vi "ESC Pre Analysis Plugin.vi"() -> ()   [LabVIEW 2022 SP3]
uses:
  <vilib>/Analysis/baseanly.llb/Mean (DBL).vi
  Globals/Meas_global.vi
  <vilib>/measure/matone.llb/Extract Single Tone Information 1 Chan.vi
  <vilib>/measure/NI_MAPro.lvlib
  <vilib>/Analysis/NI_AALBase.lvlib
panel:
  in  "Blades/Poles":i32[](array[numeric])
  in  "Freq Channels":i32[](array[numeric])
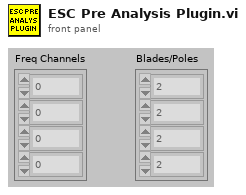
[diagram p1: front panel]
types:
  T1 = typedef "Analysis_info_cluster.ctl" = cluster{"Colour":u32, "Inst type":T2, "Inst name":string, "Symbol":string, "Code name":string, "Extra Info":string, "Inst Array":T3, "U":dbl, "u^2":dbl, "u^3":dbl, "u^4":dbl, "Skew_u":dbl, "Kurt_u":dbl, "Sd Error in Mean":dbl, "% u'/U":dbl, "X":dbl, "Y":dbl, "Z":dbl, "Timescale integral Estimate":dbl, "Sd Error in Variance":dbl, "Calib File":path, "Calib Constants":dbl[], "Output Position":bool, "Stats":enum16{"None", "Basic", "Full"}, "Av Sampling Rate":dbl, "Av No of Samples":dbl, "Total Meas Time (s)":dbl, "OrigChName":string, "Max value":dbl, "Min value":dbl, "Req Sample Rate Hz":dbl, "Sync Delay Time (s)":dbl, "Ch No":i16, "Device":string, "Use Latest Calib":bool, "Port":string, "Metadata Ch Names":string[], "Metadata Ch Values":string[], "Label":string, "chState":T4, "Point Drift":dbl, "inputConfig":string}
  T2 = typedef "Inst_type.ctl" = enum16{"Raw voltage", "Raw with zero offsetting", "Propeller anemometer", "Pressure Transducer", "Pitot-static tube", "Hot wire", "Cross wire 1", "Cross wire 2", "Generic Linear", "Generic Polynomial", "Generic BackPoly", "Fast FID", "Thermocouple", "Cold wire", "Pulsed Wire", "LDA Vel", "LDA Tran time", "LDA Arr time", "Microphone"}
  T3 = typedef "Instrument_Array.ctl" = enum16{"PWA", "LDA", "Analogue"}
  T4 = typedef "channelState.ctl" = enum32{"No Selection", "Solo", "Mute"}
  T5 = typedef "Setup.ctl" = enum16{"Run Program", "Show Setup", "Save Current Setup", "Setup Front Panel"}
  T6 = typedef "Time_Trace_Cluster.ctl" = cluster{"Weighting":dbl[], "Voltage":dbl[], "Eng Values":dbl[]}
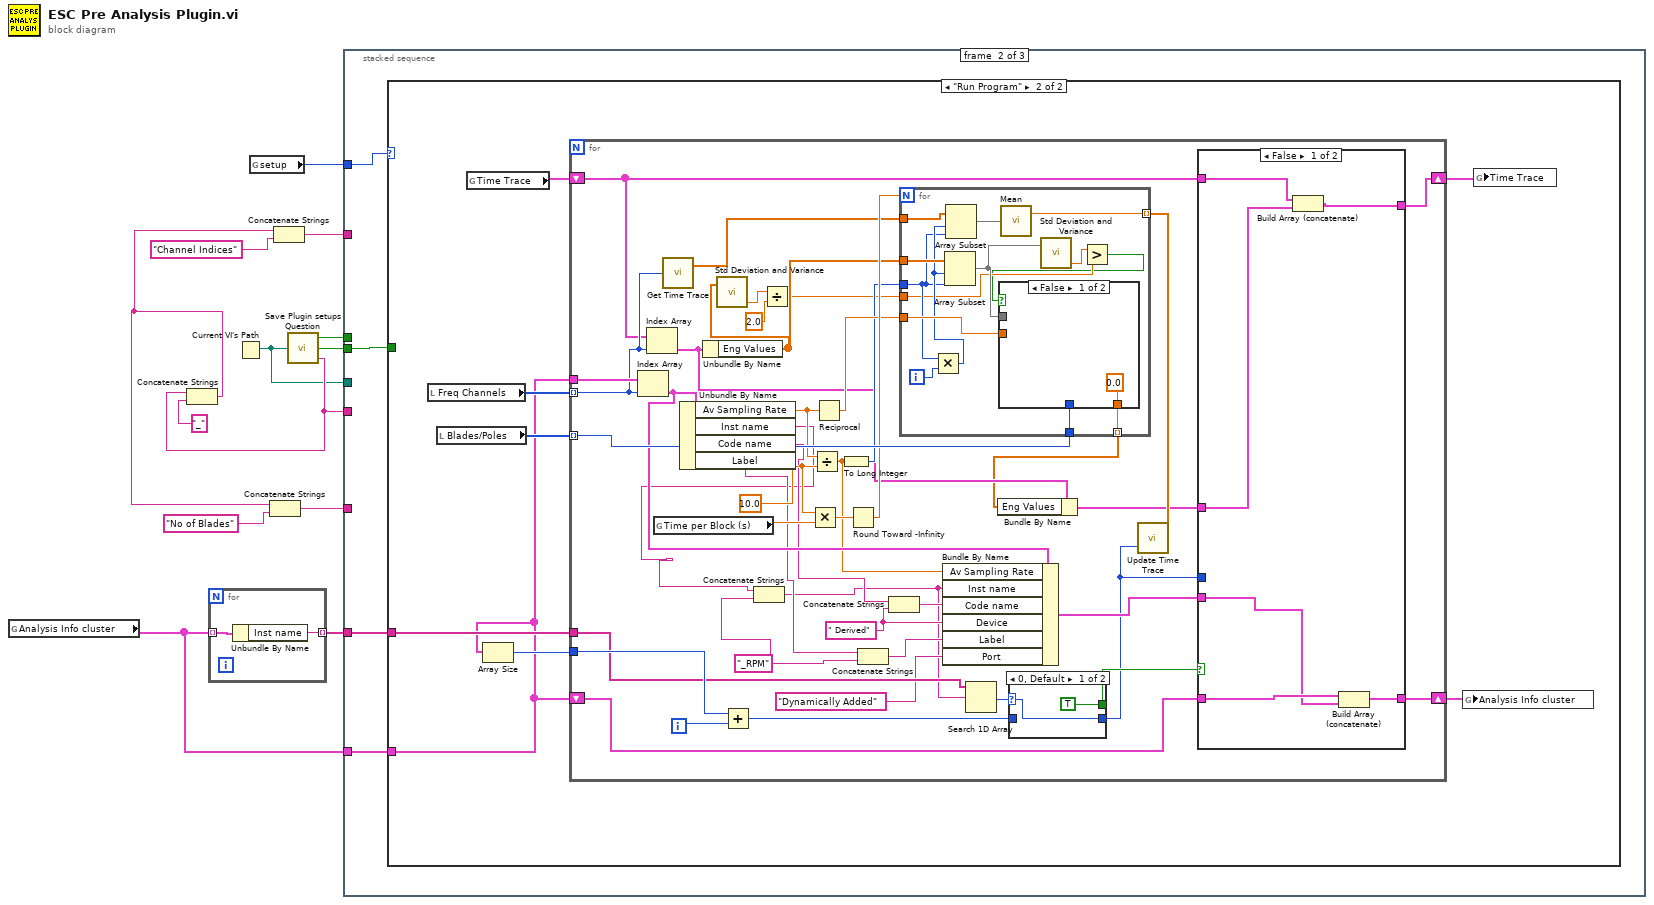
[diagram p0: block diagram]
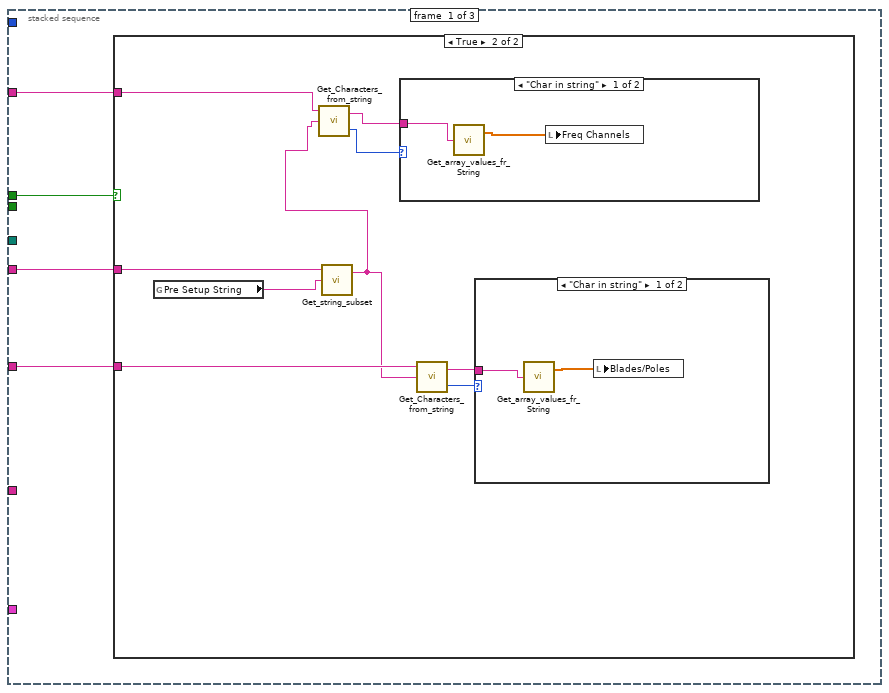
[diagram p2: hidden frame]
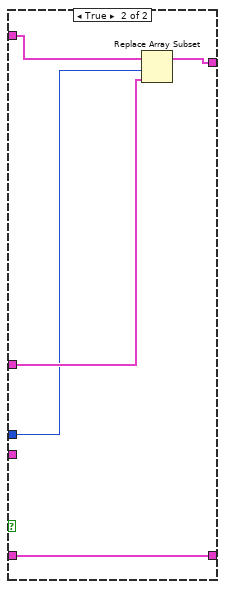
[diagram p7: hidden frame]
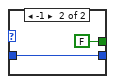
[diagram p8: hidden frame]
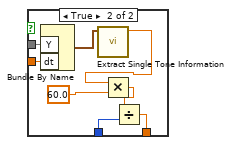
[diagram p9: hidden frame]
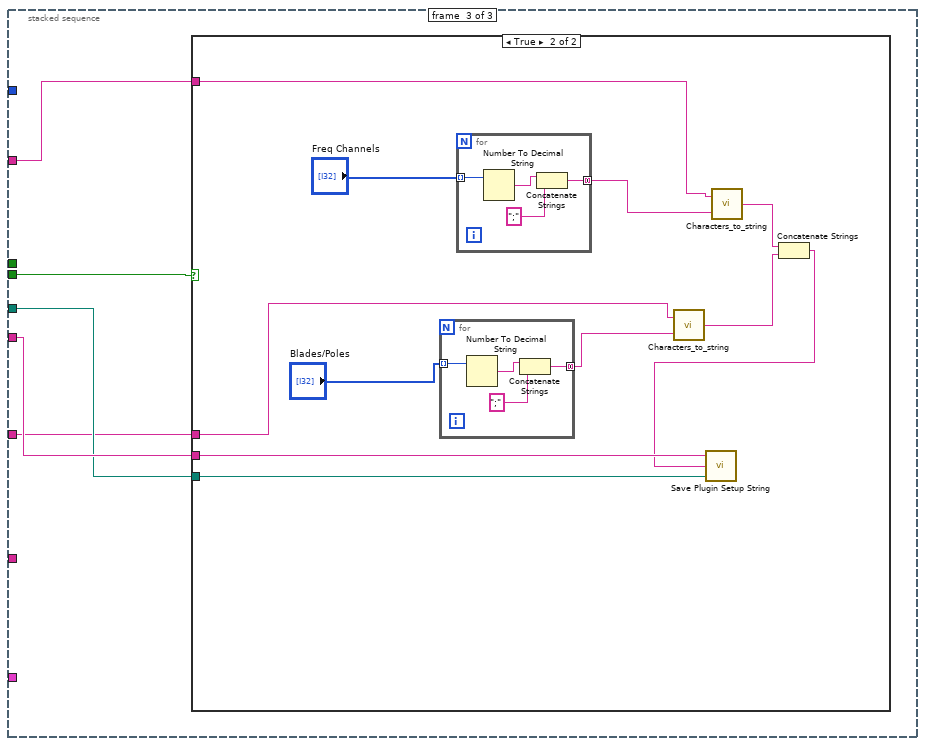
[diagram p10: hidden frame]
diagram:
  n1 = global read "Meas_global.vi" "Analysis Info cluster"() -> (w2:T1[])
  n2 = for {
    tunnel: w2 -> [w15] mode=indexing
    tunnel: [w14] -> w1 mode=indexing
    n3 = Unbundle By Name(w15) -> ("Inst name"=w14:string)
  }
  n4 = Current VI's Path() -> (path=w7:path)
  n5 = global read "Meas_global.vi" "setup"() -> (w3:T5)
  n6 = call "Save Plugin setups Question.vi"("VI path"=w7) -> ("Load Plugin Setup"=w13:bool, "Save Plugin Setup"=w8:bool, "Plugin_Label"=w9:string)
  n7 = Concatenate Strings(w9, "_" ("string")) -> (w5:string)
  n8 = Concatenate Strings(w5, "No of Blades" ("Label for value")) -> (w4:string)
  n9 = Concatenate Strings(w5, "Channel Indices" ("Label for value")) -> (w10:string)
  n10 = stacked-sequence {
    tunnel: w13 -> [w19 _ _]
    tunnel: w10 -> [w18 _ w127]
    tunnel: w9 -> [w17 _ w128]
    tunnel: w8 -> [_ w35 w129]
    tunnel: w7 -> [_ _ w126]
    tunnel: w4 -> [w16 _ w125]
    tunnel: w3 -> [_ w36 _]
    tunnel: w2 -> [_ w34 _]
    tunnel: w1 -> [_ w33 _]
    frame #0 {
      n11 = case shown="True" w19 {
        tunnel: w18 -> [_ w23]
        tunnel: w17 -> [_ w27]
        tunnel: w16 -> [_ w26]
        frame False {
        }
        frame True {
          n12 = global read "Meas_global.vi" "Pre Setup String"() -> (w28:string)
          n13 = call "Get_string_subset.vi"("String to split"=w28, "File Label"=w27) -> ("Output string"=w22:string)  [unwired: 2 in, 1 out]
          n14 = call "Get_Characters_from_string.vi"("Input string"=w22, "Variable name"=w23) -> ("Status"=w20:enum16{"Char in string", "Char not in string"}, "Value"=w21:string)  [unwired: 1 in]
          n15 = case shown="\"Char in string\"" w20 {
            tunnel: w21 -> [w32 _]
            frame "Char in string" {
              n16 = call "Get_array_values_fr_String.vi"("String Value"=w32) -> ("Numeric Array"=w31:dbl[])  [unwired: 1 out]
              n17 = local write "Freq Channels"(w31) -> ()
            }
            frame "Char not in string" {
            }
          }
          n18 = call "Get_Characters_from_string.vi"("Input string"=w22, "Variable name"=w26) -> ("Status"=w25:enum16{"Char in string", "Char not in string"}, "Value"=w24:string)  [unwired: 1 in]
          n19 = case shown="\"Char in string\"" w25 {
            tunnel: w24 -> [w30 _]
            frame "Char in string" {
              n20 = call "Get_array_values_fr_String.vi"("String Value"=w30) -> ("Numeric Array"=w29:dbl[])  [unwired: 1 out]
              n21 = local write "Blades/Poles"(w29) -> ()
            }
            frame "Char not in string" {
            }
          }
        }
      }
    }
    frame #1 {
      n22 = case shown="\"Run Program\"" w36 {
        tunnel: w35 -> [_ _]
        tunnel: w34 -> [_ w39]
        tunnel: w33 -> [_ w44]
        frame Default {
        }
        frame "Run Program" {
          n23 = local read "Freq Channels"() -> (w43:i32[])
          n24 = local read "Blades/Poles"() -> (w42:i32[])
          n25 = global read "Meas_global.vi" "Time Trace"() -> (w40:T6[])
          n26 = Array Size(array=w39) -> (size(s)=w41:i32)
          n27 = for {
            tunnel: w39 -> [w86]
            tunnel: w43 -> [w85] mode=indexing
            tunnel: w42 -> [w84] mode=indexing
            tunnel: w41 -> [w82]
            tunnel: w44 -> [w81]
            shift-right: [w57] -> w37
            shift-left: w40 -> [w59]
            shift-right: [w55] -> w38
            shift-left: w39 -> [w56]
            i -> [w83]
            w51 = " Derived" ("string")
            w48 = "_RPM" ("string")
            w78 = 10.0 ("y")
            n28 = Index Array(array=w86, index=w85) -> (element=w73:T1)
            n29 = Index Array(array=w59, index=w85) -> (element=w70:T6)
            n30 = global read "Meas_global.vi" "Time per Block (s)"() -> (w79:dbl)
            n31 = call "Get Time Trace.vi"("Channel Index"=w85) -> ("Time (s)"=w71:dbl[])  [unwired: 1 out]
            n32 = Unbundle By Name(w73) -> ("Av Sampling Rate"=w80:dbl, "Inst name"=w45:string, "Code name"=w52:string, "Label"=w50:string)
            n33 = Unbundle By Name(w70) -> ("Eng Values"=w68:dbl[])
            n34 = call <vilib>:"Std Deviation and Variance.vi"("X"=w68) -> ("variance"=w67:dbl)  [unwired: 1 in, 2 out]
            n35 = Add(x=w82, y=w83) -> (x+y=w61:i32)
            n36 = Concatenate Strings(w45, w48) -> (w46:string)
            n37 = Divide(x=w67, y=2.0) -> (x/y=w65:dbl)
            n38 = Multiply(x=w78, y=w79) -> (x*y=w77:dbl)
            n39 = Divide(x=w80, y=w78) -> (x/y=w72:dbl)
            n40 = Reciprocal(x=w80) -> (1/x=w75:dbl)
            n41 = To Long Integer(number=w72) -> (32bit integer=w74:i32)
            n42 = Round Toward -Infinity(1:w77) -> (0:w76:dbl)
            n43 = Concatenate Strings(w50, w48) -> (w49:string)
            n44 = Concatenate Strings(w52, w51) -> (w63:string)
            n45 = for {
              N: w76 -> [_]
              tunnel: w68 -> [w114]
              tunnel: w75 -> [w115]
              tunnel: w74 -> [w111]
              tunnel: w71 -> [w110]
              tunnel: [w108] -> w69 mode=indexing
              tunnel: w84 -> [w107]
              tunnel: w65 -> [w104]
              tunnel: [w102] -> w64 mode=indexing
              i -> [w113]
              n46 = Multiply(x=w111, y=w113) -> (x*y=w112:i32)
              n47 = Array Subset(array=w114, index=w112, length=w111) -> (w106:dbl[])
              n48 = Array Subset(array=w110, index=w112, length=w111) -> (w109:dbl[])
              n49 = call-poly <vilib>:"Mean.vi"("X"=w109) -> ("mean"=w108:dbl)  [unwired: 1 out]
              n50 = call <vilib>:"Std Deviation and Variance.vi"("X"=w106) -> ("variance"=w105:dbl)  [unwired: 1 in, 2 out]
              n51 = Greater?(x=w105, y=w104) -> (0:w103:bool)
              n52 = case shown="False" w103 {
                tunnel: w115 -> [_ w123]
                tunnel: w107 -> [_ w119]
                tunnel: w106 -> [_ w118]
                tunnel: [0.0 w117] -> w102
                frame False {
                }
                frame True {
                  n53 = Bundle By Name("Y"=w118, "dt"=w123) -> (w124:waveform(dbl))  [unwired: 1 in]
                  n54 = call-poly <vilib>:"Extract Single Tone Information.vi"("time signal in"=w124) -> ("detected frequency"=w120:dbl)  [unwired: 5 in, 5 out]
                  n55 = Multiply(x=w120, y=60.0) -> (x*y=w121:dbl)
                  n56 = Divide(x=w121, y=w119) -> (x/y=w117:dbl)
                }
              }
            }
            n57 = Bundle By Name(cluster=w73, "Av Sampling Rate"=w72, "Inst name"=w46, "Code name"=w63, "Device"=w51, "Label"=w49, "Port"="Dynamically Added") -> (w54:T1)
            n58 = Search 1D Array(1D array=w81, element=w46) -> (index of element=w62:i32)  [unwired: 1 in]
            n59 = Bundle By Name(cluster=w70, "Eng Values"=w64) -> (w58:T6)
            n60 = case shown="0, Default" w62 {
              selector: w62 -> [w99 _]
              tunnel: [w99 w101] -> w53
              tunnel: w61 -> [_ w101]
              tunnel: [TRUE FALSE] -> w60
              frame 0, Default {
              }
              frame -1 {
              }
            }
            n61 = call "Update Time Trace.vi"("Channel Index"=w53, "Time (s)"=w69) -> ()  [unwired: 1 in]
            n62 = case shown="False" w60 {
              tunnel: w59 -> [w92 w97]
              tunnel: w58 -> [w91 w95]
              tunnel: [w90 w96] -> w57
              tunnel: w56 -> [w89 w93]
              tunnel: [w88 w93] -> w55
              tunnel: w54 -> [w87 _]
              tunnel: w53 -> [_ w94]
              frame False {
                n63 = Build Array (concatenate)(w92, w91) -> (w90:T6[])
                n64 = Build Array (concatenate)(w89, w87) -> (w88:T1[])
              }
              frame True {
                n65 = Replace Array Subset(array=w97, new element=w95, index=w94) -> (w96:T6[])
              }
            }
          }
          n66 = global write "Meas_global.vi" "Analysis Info cluster"(w38) -> ()
          n67 = global write "Meas_global.vi" "Time Trace"(w37) -> ()
        }
      }
    }
    frame #2 {
      n68 = case shown="True" w129 {
        tunnel: w128 -> [_ w140]
        tunnel: w127 -> [_ w137]
        tunnel: w126 -> [_ w139]
        tunnel: w125 -> [_ w133]
        frame False {
        }
        frame True {
          n69 = for {
            tunnel: "Blades/Poles" -> [w144] mode=indexing
            tunnel: [w141] -> w132 mode=concatenating
            n70 = Number To Decimal String(number=w144) -> (decimal integer string=w143:string)  [unwired: 1 in]
            n71 = Concatenate Strings(w143, ";") -> (w141:string)
          }
          n72 = for {
            tunnel: "Freq Channels" -> [w148] mode=indexing
            tunnel: [w145] -> w136 mode=concatenating
            n73 = Number To Decimal String(number=w148) -> (decimal integer string=w147:string)  [unwired: 1 in]
            n74 = Concatenate Strings(w147, ";") -> (w145:string)
          }
          n75 = call "Characters_to_string.vi"("Characters to write"=w132, "Label for characters"=w133) -> ("Output string"=w131:string)  [unwired: 1 in]
          n76 = call "Characters_to_string.vi"("Characters to write"=w136, "Label for characters"=w137) -> ("Output string"=w135:string)  [unwired: 1 in]
          n77 = Concatenate Strings(w135, w131) -> (w138:string)
          n78 = call "Save Plugin Setup String.vi"("Plug In Pathname"=w139, "Setup String to Save"=w138, "PlugIn Label"=w140) -> ()  [unwired: 2 out]
        }
      }
    }
  }
